vi "Change file locations.vi"(8 "Error In":errorcluster, 11 "INI ref in":T1) -> (0 "Error Out":errorcluster, 3 "INI ref out":T1)   [LabVIEW 2015]
uses:
  <vilib>/Utility/config.llb/Config Data RefNum.ctl
  Create destinations/Change files state.ctl
  <vilib>/Utility/sysdir.llb/System Directory Type.ctl
  <vilib>/Utility/config.llb/Write Key (Boolean).vi
  <vilib>/Utility/config.llb/Write Key (Path).vi
  <vilib>/Utility/config.llb/Read Key (Path).vi
  <vilib>/Utility/config.llb/NI_LVConfig.lvlib
panel:
  in  "Create folder":bool
  out "Success":string caption="Config Message"
  in  "Open":bool
  in  "Cancel":bool
  in  "Update":bool
  in  "Folder path":path
  in  "File types":enum16{"Data Files", "Record Files"}(ring)
  # "Change file locations\n\nPlease select the folder that contains the files, and then click Update paths. You will be prompted to create them automatically if they do not exist."
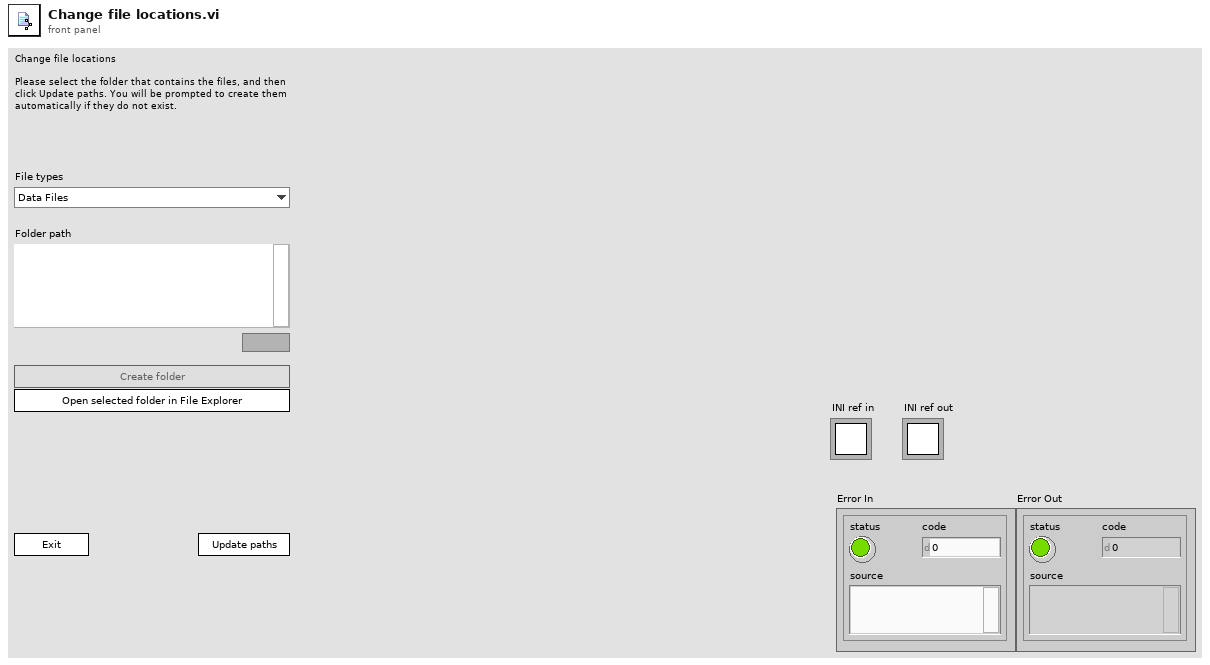
[diagram p1: front panel]
types:
  T1 = typedef "NI_LVConfig.lvlib/Config Data RefNum.ctl" = refnum<k1>
  T2 = typedef "Change files state.ctl" = enum16{"Init", "Idle", "Edit data path", "Edit records path", "Open folder", "Exit"}
  T3 = enum8{"Enabled", "Disabled", "Disabled and Grayed Out"}
  T4 = enum16{"open", "replace", "create", "open or create", "replace or create", "replace or create with confirmation"}
  T5 = typedef "System Directory Type.ctl" = i32
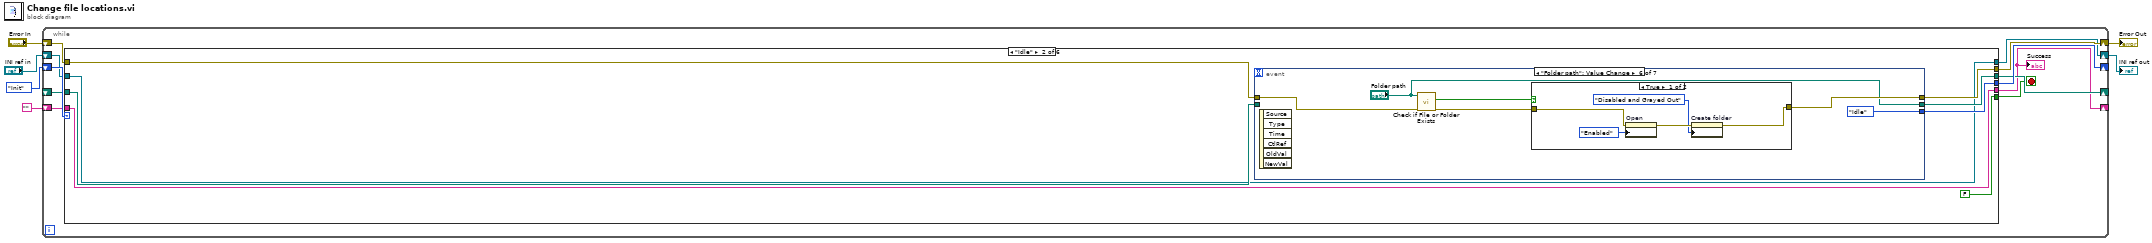
[diagram p0: block diagram]
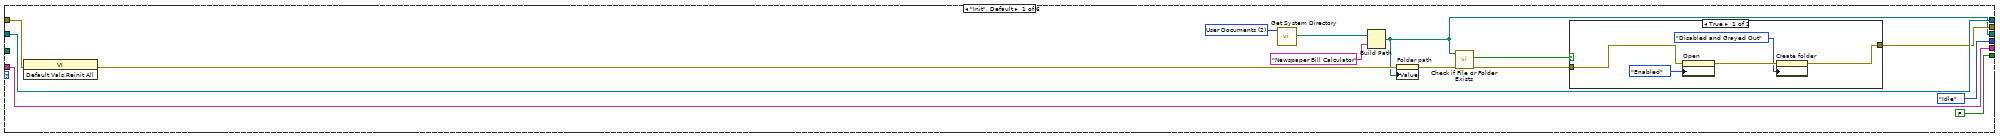
[diagram p2: hidden frame]
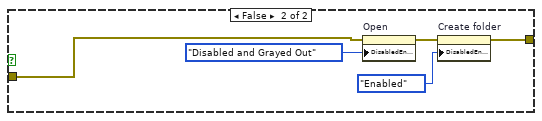
[diagram p3: hidden frame]
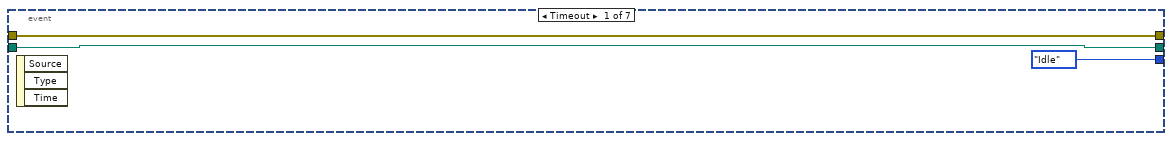
[diagram p4: hidden frame]
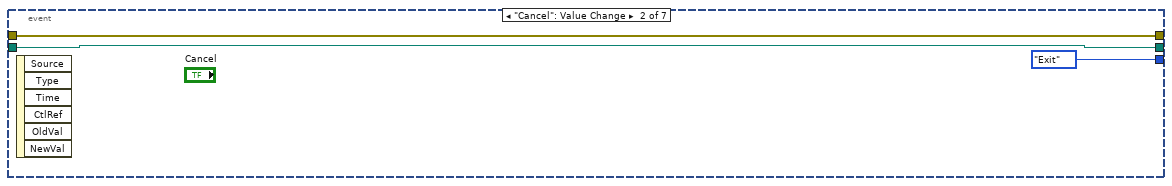
[diagram p5: hidden frame]
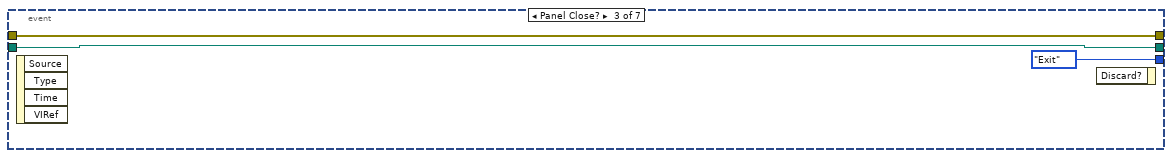
[diagram p6: hidden frame]
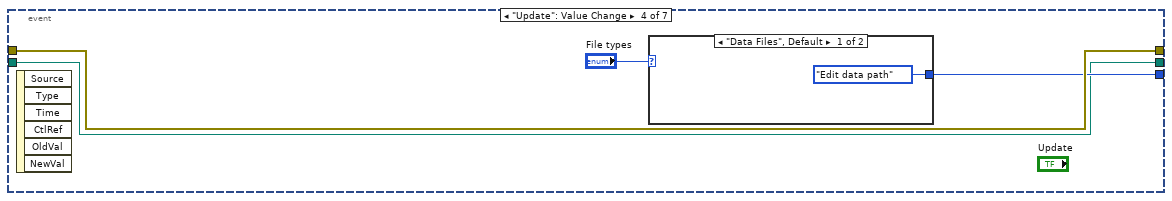
[diagram p7: hidden frame]
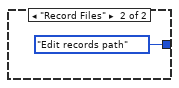
[diagram p8: hidden frame]
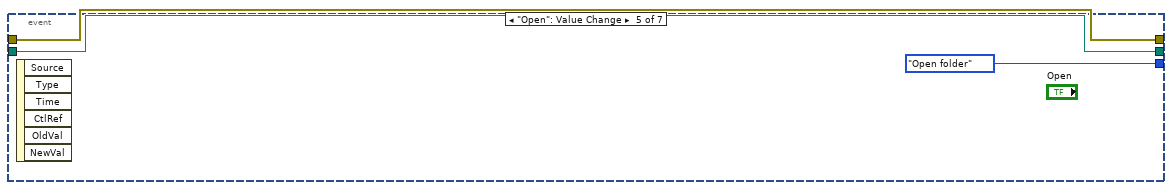
[diagram p9: hidden frame]
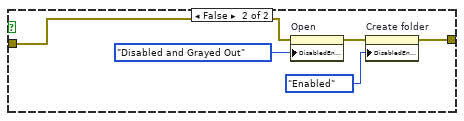
[diagram p10: hidden frame]
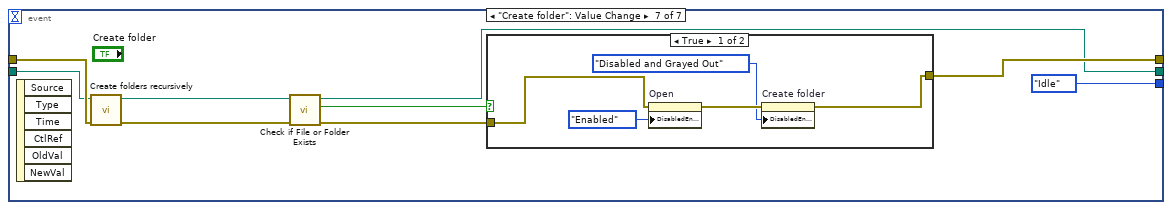
[diagram p11: hidden frame]
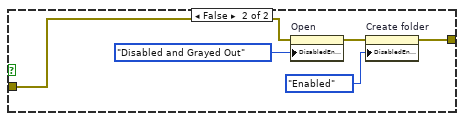
[diagram p12: hidden frame]
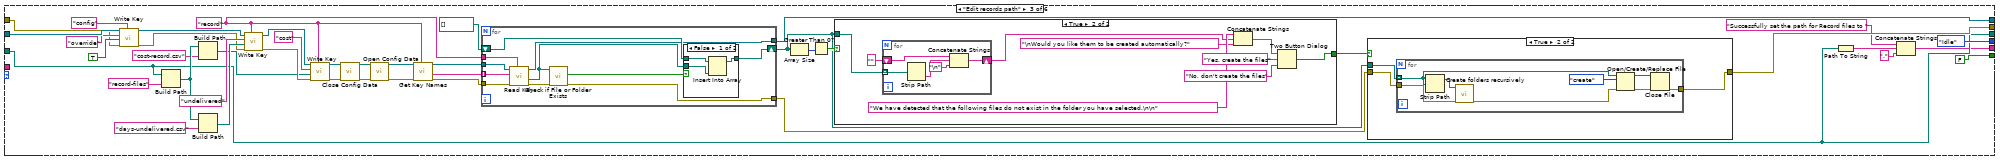
[diagram p13: hidden frame]
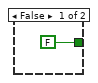
[diagram p15: hidden frame]
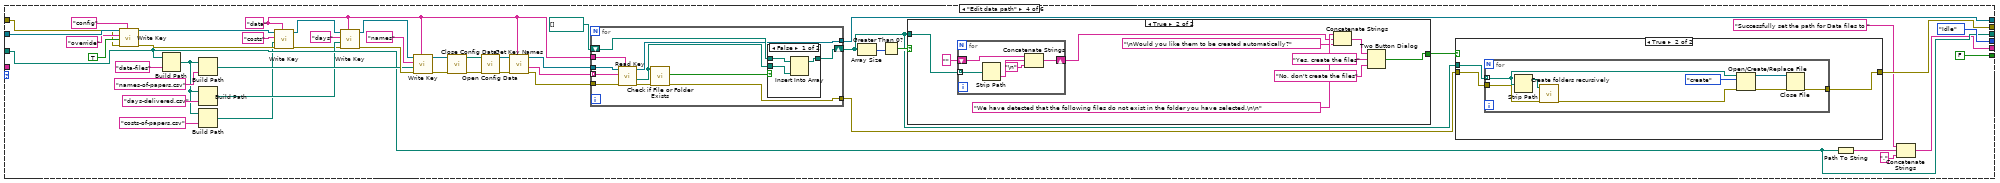
[diagram p17: hidden frame]
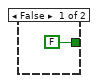
[diagram p19: hidden frame]
diagram:
  n1 = while {
    shift-right: [w16] -> _
    shift-left: Change_files_state."Init" -> [w17]
    shift-right: [w14] -> w4
    shift-left: "Error In" -> [w15]
    shift-right: [w12] -> _
    shift-left: _ -> [w11]
    shift-right: [w10] -> w2
    shift-left: "INI ref in" -> [w13]
    shift-right: [w9] -> _
    shift-left: "" -> [w8]
    stop <- w7 stop-if-true
    n2 = case shown="\"Idle\"" w17 {
      tunnel: [Change_files_state."Idle" w49 Change_files_state."Idle" Change_files_state."Idle" Change_files_state."Idle" Change_files_state."Exit"] -> w16
      tunnel: w15 -> [w27 w47 w110 w204 w282 w287]
      tunnel: [w20 w48 w123 w214 w278 w287] -> w14
      tunnel: [FALSE FALSE FALSE FALSE FALSE TRUE] -> w7
      tunnel: w13 -> [w25 w43 w141 w230 w281 w288]
      tunnel: [w19 w46 w120 w211 w276 w286] -> w12
      tunnel: w11 -> [_ w45 w120 w211 w276 w286]
      tunnel: [w25 w43 w116 w187 w281 w288] -> w10
      tunnel: [w24 w42 w118 w209 w277 w285] -> w9
      tunnel: w8 -> [w24 w42 _ _ w277 w285]
      frame "Init", Default {
        w30 = T5 2 items=["User Home"=0, "User Desktop"=1, "User Documents"=2, "User Application Data"=3, "User Preferences"=4, "User Temporary"=5, "Public Documents"=6, "Public Application Data"=7, "Public Preferences"=8, "Public Cache"=13, "System Core Libraries"=9, "System Installed Libraries"=10, "Application Files"=11, "Boot Volume Root"=12] ("system directory type")
        n3 = invoke class="VI" method="Default Vals.Reinit All"(error in=w27) -> (error out=w23:errorcluster)  [unwired: 2 in, 2 out]
        n4 = call <vilib>:"Get System Directory.vi"("system directory type"=w30) -> ("system directory"=w29:path)  [unwired: 10 in]
        n5 = Build Path(base path=w29, name or relative path="Newspaper Bill Calculator") -> (appended path=w19:path)
        n6 = property on="Folder path" class="Path"(error in=w23, "Value"=w19) -> (error out=w22:errorcluster)  [unwired: 1 in, 1 out]
        n7 = call <vilib>:"Check if File or Folder Exists.vi"("error in (no error)"=w22, "path"=w19) -> ("error out"=w21:errorcluster, "file or folder exists?"=w18:bool)  [unwired: 7 in, 1 out]
        n8 = case shown="True" w18 {
          tunnel: w21 -> [w36 w41]
          tunnel: [w34 w39] -> w20
          frame True {
            n9 = property on="Open" class="Bool"(error in=w36, "DisabledEnum"=T3."Enabled" ("Disabled")) -> (error out=w35:errorcluster)  [unwired: 1 in, 1 out]
            n10 = property on="Create folder" class="Bool"(error in=w35, "DisabledEnum"=T3."Disabled and Grayed Out" ("Disabled")) -> (error out=w34:errorcluster)  [unwired: 1 in, 1 out]
          }
          frame False {
            n11 = property on="Open" class="Bool"(error in=w41, "DisabledEnum"=T3."Disabled and Grayed Out" ("Disabled")) -> (error out=w40:errorcluster)  [unwired: 1 in, 1 out]
            n12 = property on="Create folder" class="Bool"(error in=w40, "DisabledEnum"=T3."Enabled" ("Disabled")) -> (error out=w39:errorcluster)  [unwired: 1 in, 1 out]
          }
        }
      }
      frame "Idle" {
        n13 = event shown="[5] \"Folder path\": Value Change" {
          selector: _ -> [_ _ _ _ _ _ _]
          dyn-events: _ -> [_ _ _ _ _ _ _]
          timeout: _ -> [_ _ _ _ _ _ _]
          tunnel: [Change_files_state."Idle" Change_files_state."Exit" Change_files_state."Exit" w60 Change_files_state."Open folder" Change_files_state."Idle" Change_files_state."Idle"] -> w49
          tunnel: [w51 w54 w57 w62 w66 w69 w90] -> w48
          tunnel: w47 -> [w51 w54 w57 w62 w66 w73 w86]
          tunnel: [w50 w53 w56 w59 w65 "Folder path" w87] -> w46
          tunnel: w45 -> [w50 w53 w56 w59 w65 _ w84]
          event Timeout {
            n14 = event-data() -> ()  [unwired: 1 in, 3 out]
          }
          event "Cancel": Value Change {
            n15 = event-data() -> ()  [unwired: 1 in, 6 out]
          }
          event Panel Close? {
            n16 = event-data() -> ()  [unwired: 1 in, 4 out]
            n17 = event-data() -> ()  [unwired: 2 in, 1 out]
          }
          event "Update": Value Change {
            n18 = event-data() -> ()  [unwired: 1 in, 6 out]
            n19 = case shown="\"Data Files\", Default" "File types" {
              tunnel: [Change_files_state."Edit data path" Change_files_state."Edit records path"] -> w60
              frame "Data Files", Default {
              }
              frame "Record Files" {
              }
            }
          }
          event "Open": Value Change {
            n20 = event-data() -> ()  [unwired: 1 in, 6 out]
          }
          event "Folder path": Value Change {
            n21 = event-data() -> ()  [unwired: 1 in, 6 out]
            n22 = call <vilib>:"Check if File or Folder Exists.vi"("error in (no error)"=w73, "path"="Folder path") -> ("error out"=w71:errorcluster, "file or folder exists?"=w70:bool)  [unwired: 7 in, 1 out]
            n23 = case shown="True" w70 {
              tunnel: w71 -> [w78 w83]
              tunnel: [w76 w81] -> w69
              frame True {
                n24 = property on="Open" class="Bool"(error in=w78, "DisabledEnum"=T3."Enabled" ("Disabled")) -> (error out=w77:errorcluster)  [unwired: 1 in, 1 out]
                n25 = property on="Create folder" class="Bool"(error in=w77, "DisabledEnum"=T3."Disabled and Grayed Out" ("Disabled")) -> (error out=w76:errorcluster)  [unwired: 1 in, 1 out]
              }
              frame False {
                n26 = property on="Open" class="Bool"(error in=w83, "DisabledEnum"=T3."Disabled and Grayed Out" ("Disabled")) -> (error out=w82:errorcluster)  [unwired: 1 in, 1 out]
                n27 = property on="Create folder" class="Bool"(error in=w82, "DisabledEnum"=T3."Enabled" ("Disabled")) -> (error out=w81:errorcluster)  [unwired: 1 in, 1 out]
              }
            }
          }
          event "Create folder": Value Change {
            n28 = event-data() -> ()  [unwired: 1 in, 6 out]
            n29 = call "Create folders recursively.vi"("error in (no error)"=w86, "Path in"=w84) -> ("error out"=w85:errorcluster, "Path out"=w88:path)  [unwired: 8 in]
            n30 = call <vilib>:"Check if File or Folder Exists.vi"("error in (no error)"=w85, "path"=w88) -> ("error out"=w92:errorcluster, "file or folder exists?"=w91:bool, "dup path"=w87:path)  [unwired: 7 in]
            n31 = case shown="True" w91 {
              tunnel: w92 -> [w97 w102]
              tunnel: [w95 w100] -> w90
              frame True {
                n32 = property on="Open" class="Bool"(error in=w97, "DisabledEnum"=T3."Enabled" ("Disabled")) -> (error out=w96:errorcluster)  [unwired: 1 in, 1 out]
                n33 = property on="Create folder" class="Bool"(error in=w96, "DisabledEnum"=T3."Disabled and Grayed Out" ("Disabled")) -> (error out=w95:errorcluster)  [unwired: 1 in, 1 out]
              }
              frame False {
                n34 = property on="Open" class="Bool"(error in=w102, "DisabledEnum"=T3."Disabled and Grayed Out" ("Disabled")) -> (error out=w101:errorcluster)  [unwired: 1 in, 1 out]
                n35 = property on="Create folder" class="Bool"(error in=w101, "DisabledEnum"=T3."Enabled" ("Disabled")) -> (error out=w100:errorcluster)  [unwired: 1 in, 1 out]
              }
            }
          }
        }
      }
      frame "Edit records path" {
        w117 = "record" ("section")
        n36 = call-poly <vilib>:"Write Key.vi"("section"="config", "error in (no error)"=w110, "value"=TRUE, "key"="override", "refnum"=w141) -> ("error out"=w109:errorcluster, "refnum out"=w114:T1)  [unwired: 4 in, 1 out]
        n37 = Build Path(base path=w120, name or relative path="record-files") -> (appended path=w134:path)
        n38 = Build Path(base path=w134, name or relative path="cost-record.csv") -> (appended path=w135:path)
        n39 = Build Path(base path=w134, name or relative path="days-undelivered.csv") -> (appended path=w136:path)
        n40 = call-poly <vilib>:"Write Key.vi"("section"=w117, "error in (no error)"=w109, "value"=w136, "key"="undelivered" ("section"), "refnum"=w114) -> ("error out"=w139:errorcluster, "refnum out"=w138:T1)  [unwired: 4 in, 1 out]
        n41 = call-poly <vilib>:"Write Key.vi"("section"=w117, "error in (no error)"=w139, "value"=w135, "key"="cost", "refnum"=w138) -> ("error out"=w104:errorcluster, "refnum out"=w103:T1)  [unwired: 4 in, 1 out]
        n42 = call <vilib>:"Close Config Data.vi"("error in (no error)"=w104, "refnum"=w103) -> ("error out"=w106:errorcluster, "file path"=w105:path)  [unwired: 8 in]
        n43 = call <vilib>:"Open Config Data.vi"("error in (no error)"=w106, "configuration file path"=w105) -> ("error out"=w108:errorcluster, "refnum"=w107:T1)  [unwired: 7 in, 1 out]
        n44 = call <vilib>:"Get Key Names.vi"("section"=w117, "error in (no error)"=w108, "refnum"=w107) -> ("error out"=w129:errorcluster, "key names"=w131:string[], "refnum out"=w130:T1)  [unwired: 5 in, 1 out]
        n45 = for {
          tunnel: w131 -> [w182] mode=indexing
          tunnel: w130 -> [w181]
          tunnel: w129 -> [w180]
          shift-right: [w177] -> w124
          shift-left: path[] [] -> [w178]
          tunnel: [w174] -> w116
          tunnel: [w173] -> w115
          tunnel: w117 -> [w172]
          n46 = call-poly <vilib>:"Read Key.vi"("section"=w172, "error in (no error)"=w180, "key"=w182, "refnum"=w181) -> ("error out"=w179:errorcluster, "value"=w176:path, "refnum out"=w174:T1)  [unwired: 4 in, 1 out]
          n47 = call <vilib>:"Check if File or Folder Exists.vi"("error in (no error)"=w179, "path"=w176) -> ("error out"=w173:errorcluster, "file or folder exists?"=w175:bool)  [unwired: 7 in, 1 out]
          n48 = case shown="False" w175 {
            tunnel: w178 -> [w185 w186]
            tunnel: [w184 w186] -> w177
            tunnel: w176 -> [w183 _]
            frame False {
              n49 = Insert Into Array(array=w185, new element=w183) -> (w184:path[])  [unwired: 1 in]
            }
            frame True {
            }
          }
        }
        n50 = Array Size(array=w124) -> (size(s)=w127:i32)
        n51 = Greater Than 0?(x=w127) -> (x > 0?=w126:bool)
        n52 = case shown="True" w126 {
          tunnel: w124 -> [_ w166]
          tunnel: [FALSE ("T button?") w158] -> w125
          frame False {
          }
          frame True {
            n53 = for {
              tunnel: w166 -> [w171] mode=indexing
              shift-right: [w170] -> w163
              shift-left: "" -> [w169]
              n54 = Strip Path(path=w171) -> (name=w168:string)  [unwired: 1 out]
              n55 = Concatenate Strings(w169, w168, "\n") -> (w170:string)
            }
            n56 = Concatenate Strings("We have detected that the following files do not exist in the folder you have selected.\n\n" ("string"), w163, "\nWould you like them to be created automatically?" ("string")) -> (w161:string)
            n57 = Two Button Dialog(message=w161, 1:"No, don't create the files" ("F button name (\"Cancel\")"), 2:"Yes, create the files" ("T button name (\"OK\")")) -> (T button?=w158:bool)
          }
        }
        n58 = case shown="True" w125 {
          tunnel: w124 -> [_ w148]
          tunnel: w115 -> [w145 w147]
          tunnel: [w145 w146] -> w123
          frame False {
          }
          frame True {
            n59 = for {
              tunnel: w148 -> [w149] mode=indexing
              tunnel: w147 -> [w151]
              tunnel: [w153] -> w146
              n60 = Strip Path(path=w149) -> (stripped path=w152:path)  [unwired: 1 out]
              n61 = call "Create folders recursively.vi"("error in (no error)"=w151, "Path in"=w152) -> ("error out"=w150:errorcluster)  [unwired: 8 in, 1 out]
              n62 = Open/Create/Replace File(file path (use dialog)=w149, error in=w150, operation (0:open)=T4."create") -> (refnum out=w155:refnum<file>, error out=w156:errorcluster)  [unwired: 3 in, 1 out]
              n63 = Close File(refnum=w155, error in=w156) -> (error out=w153:errorcluster)  [unwired: 1 out]
            }
          }
        }
        n64 = Path To String(path=w120) -> (string=w121:string)
        n65 = Concatenate Strings("Successfully set the path for Record files to " ("string"), w121, "." ("string")) -> (w118:string)
      }
      frame "Edit data path" {
        w196 = "data" ("section")
        n66 = call-poly <vilib>:"Write Key.vi"("section"="config", "error in (no error)"=w204, "value"=TRUE, "key"="override", "refnum"=w230) -> ("error out"=w197:errorcluster, "refnum out"=w198:T1)  [unwired: 4 in, 1 out]
        n67 = Build Path(base path=w211, name or relative path="data-files") -> (appended path=w202:path)
        n68 = Build Path(base path=w202, name or relative path="names-of-papers.csv") -> (appended path=w225:path)
        n69 = Build Path(base path=w202, name or relative path="days-delivered.csv") -> (appended path=w201:path)
        n70 = Build Path(base path=w202, name or relative path="costs-of-papers.csv") -> (appended path=w194:path)
        n71 = call-poly <vilib>:"Write Key.vi"("section"=w196, "error in (no error)"=w197, "value"=w194, "key"="costs", "refnum"=w198) -> ("error out"=w200:errorcluster, "refnum out"=w199:T1)  [unwired: 4 in, 1 out]
        n72 = call-poly <vilib>:"Write Key.vi"("section"=w196, "error in (no error)"=w200, "value"=w201, "key"="days" ("section"), "refnum"=w199) -> ("error out"=w228:errorcluster, "refnum out"=w227:T1)  [unwired: 4 in, 1 out]
        n73 = call-poly <vilib>:"Write Key.vi"("section"=w196, "error in (no error)"=w228, "value"=w225, "key"="names", "refnum"=w227) -> ("error out"=w193:errorcluster, "refnum out"=w192:T1)  [unwired: 4 in, 1 out]
        n74 = call <vilib>:"Close Config Data.vi"("error in (no error)"=w193, "refnum"=w192) -> ("error out"=w191:errorcluster, "file path"=w190:path)  [unwired: 8 in]
        n75 = call <vilib>:"Open Config Data.vi"("error in (no error)"=w191, "configuration file path"=w190) -> ("error out"=w189:errorcluster, "refnum"=w188:T1)  [unwired: 7 in, 1 out]
        n76 = call <vilib>:"Get Key Names.vi"("section"=w196, "error in (no error)"=w189, "refnum"=w188) -> ("error out"=w220:errorcluster, "key names"=w222:string[], "refnum out"=w221:T1)  [unwired: 5 in, 1 out]
        n77 = for {
          tunnel: w222 -> [w271] mode=indexing
          tunnel: w221 -> [w270]
          tunnel: w220 -> [w269]
          shift-right: [w266] -> w215
          shift-left: path[] [] -> [w267]
          tunnel: [w263] -> w187
          tunnel: [w262] -> w208
          tunnel: w196 -> [w261]
          n78 = call-poly <vilib>:"Read Key.vi"("section"=w261, "error in (no error)"=w269, "key"=w271, "refnum"=w270) -> ("error out"=w268:errorcluster, "value"=w265:path, "refnum out"=w263:T1)  [unwired: 4 in, 1 out]
          n79 = call <vilib>:"Check if File or Folder Exists.vi"("error in (no error)"=w268, "path"=w265) -> ("error out"=w262:errorcluster, "file or folder exists?"=w264:bool)  [unwired: 7 in, 1 out]
          n80 = case shown="False" w264 {
            tunnel: w267 -> [w274 w275]
            tunnel: [w273 w275] -> w266
            tunnel: w265 -> [w272 _]
            frame False {
              n81 = Insert Into Array(array=w274, new element=w272) -> (w273:path[])  [unwired: 1 in]
            }
            frame True {
            }
          }
        }
        n82 = Array Size(array=w215) -> (size(s)=w218:i32)
        n83 = Greater Than 0?(x=w218) -> (x > 0?=w217:bool)
        n84 = case shown="True" w217 {
          tunnel: w215 -> [_ w255]
          tunnel: [FALSE ("T button?") w247] -> w216
          frame False {
          }
          frame True {
            n85 = for {
              tunnel: w255 -> [w260] mode=indexing
              shift-right: [w259] -> w252
              shift-left: "" -> [w258]
              n86 = Strip Path(path=w260) -> (name=w257:string)  [unwired: 1 out]
              n87 = Concatenate Strings(w258, w257, "\n") -> (w259:string)
            }
            n88 = Concatenate Strings("We have detected that the following files do not exist in the folder you have selected.\n\n" ("string"), w252, "\nWould you like them to be created automatically?" ("string")) -> (w250:string)
            n89 = Two Button Dialog(message=w250, 1:"No, don't create the files" ("F button name (\"Cancel\")"), 2:"Yes, create the files" ("T button name (\"OK\")")) -> (T button?=w247:bool)
          }
        }
        n90 = case shown="True" w216 {
          tunnel: w215 -> [_ w237]
          tunnel: w208 -> [w234 w236]
          tunnel: [w234 w235] -> w214
          frame False {
          }
          frame True {
            n91 = for {
              tunnel: w237 -> [w238] mode=indexing
              tunnel: w236 -> [w240]
              tunnel: [w242] -> w235
              n92 = Strip Path(path=w238) -> (stripped path=w241:path)  [unwired: 1 out]
              n93 = call "Create folders recursively.vi"("error in (no error)"=w240, "Path in"=w241) -> ("error out"=w239:errorcluster)  [unwired: 8 in, 1 out]
              n94 = Open/Create/Replace File(file path (use dialog)=w238, error in=w239, operation (0:open)=T4."create") -> (refnum out=w244:refnum<file>, error out=w245:errorcluster)  [unwired: 3 in, 1 out]
              n95 = Close File(refnum=w244, error in=w245) -> (error out=w242:errorcluster)  [unwired: 1 out]
            }
          }
        }
        n96 = Path To String(path=w211) -> (string=w212:string)
        n97 = Concatenate Strings("Successfully set the path for Data files to " ("string"), w212, "." ("string")) -> (w209:string)
      }
      frame "Open folder" {
        n98 = call <vilib>:"System Exec.vi"("error in (no error)"=w282, "working directory"=w276, "command line"="explorer .") -> ("error out"=w278:errorcluster)  [unwired: 5 in, 3 out]
      }
      frame "Exit" {
      }
    }
    "Success" <- w9
  }
  "INI ref out" <- w2
  "Error Out" <- w4
